vi "Resynchronization Init.vi"(8 "error in":errorcluster, 11 "SCADA in":refnum<class "EMS.lvclass">) -> (0 "error out":errorcluster, 3 "SCADA out":refnum<class "EMS.lvclass">)   [LabVIEW 2018, in "EMS Core.lvlib" / "EMS.lvclass"]
uses:
  EMS.lvclass
  C:/Program Files (x86)/National Instruments/LabVIEW 2018/vi.lib/ActorFramework/Actor/Actor.lvclass
  Controls/Microgrid State.ctl
  EMS.lvclass/EMS.ctl
  <vilib>/ActorFramework/Actor/Actor.lvclass/Actor.ctl
  <vilib>/ActorFramework/Message Enqueuer/Message Enqueuer.lvclass/Message Enqueuer.ctl
  EMS Messages/Return Microgrid State Msg/Return Microgrid State Msg.lvclass/Return Microgrid State Msg.ctl
  <vilib>/ActorFramework/Message Enqueuer/Enqueue.vi
  <vilib>/ActorFramework/Stop Msg/Stop Msg.lvclass
  C:/Program Files (x86)/National Instruments/LabVIEW 2018/vi.lib/ActorFramework/Message/Message.lvclass
  EMS Messages/Return Microgrid State Msg/Return Microgrid State Msg.lvclass
  <vilib>/ActorFramework/Message Priority Queue/Priority Enqueue.vi
  <vilib>/ActorFramework/Actor/Actor.lvclass
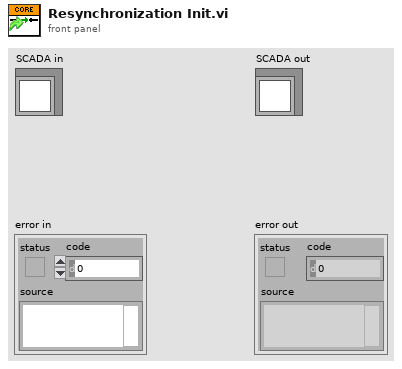
[diagram p1: front panel]
types:
  T1 = typedef "EMS Core.lvlib/EMS.lvclass/Microgrid State.ctl" = enum16{"Discovery", "Commissioning", "Activation", "Blackstart", "OnGrid", "OffGrid", "Island", "Resynchronization", "Manual", "Shutdown", "Stop"}
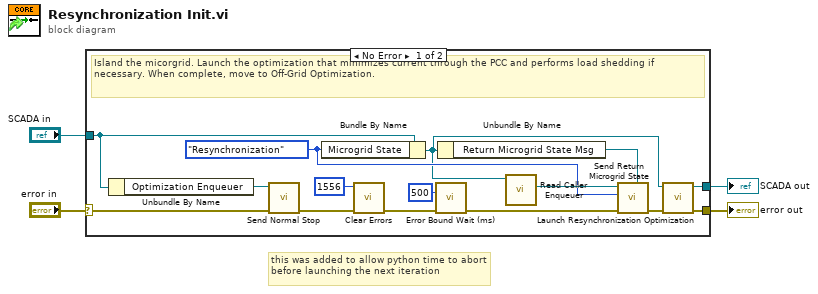
[diagram p0: block diagram]
diagram:
  # "this was added to allow python time to abort before launching the next iteration"
  n1 = case shown="No Error" "error in" {
    selector: "error in" -> [w14 w21]
    tunnel: [w10 w21] -> w3
    tunnel: [w11 w20] -> w1
    tunnel: "SCADA in" -> [w16 w20]
    frame No Error {
      w17 = Microgrid_State."Resynchronization" ("Microgrid State")
      # "Island the micorgrid. Launch the optimization that minimizes current through the PCC and performs load shedding if necessary. When complete, move to Off-Grid Optimization."
      n2 = Unbundle By Name(w16) -> ("Optimization Enqueuer"=w15:refnum<class "Message Enqueuer.lvclass">)
      n3 = call <vilib>:"Send Normal Stop.vi"("error in (no error)"=w14, "Message Enqueuer"=w15) -> ("error out"=w13:errorcluster)  [unwired: 9 in]
      n4 = Bundle By Name(cluster=w16, "Microgrid State"=w17) -> (w12:refnum<class "EMS.lvclass">)
      n5 = call <vilib>:"Clear Errors.vi"("error in (no error)"=w13, "specific error code to clear (0: all)"=1556) -> ("error out"=w8:errorcluster)  [unwired: 4 in, 1 out]
      n6 = call "Error Bound Wait (ms).vi"("milliseconds to wait (100)"=u32 500 ("milliseconds to wait"), "error in"=w8) -> ("error out"=w6:errorcluster)  [unwired: 9 in]
      n7 = Unbundle By Name(w12) -> ("Return Microgrid State Msg"=w18:refnum<class "Return Microgrid State Msg.lvclass">)
      n8 = call <vilib>:"Read Caller Enqueuer.vi"("Actor"=w12) -> ("Caller Enqueuer"=w19:refnum<class "Message Enqueuer.lvclass">)  [unwired: 10 in]
      n9 = call "Send Return Microgrid State.vi"("Message Type"=w18, "error in (no error)"=w6, "Microgrid State"=w17, "Message Enqueuer"=w19) -> ("error out"=w9:errorcluster)  [unwired: 6 in, 1 out]
      n10 = call "Launch Resynchronization Optimization.vi"("error in"=w9, "SCADA in"=w12) -> ("error out"=w10:errorcluster, "SCADA out"=w11:refnum<class "EMS.lvclass">)  [unwired: 8 in]
    }
    frame Error {
    }
  }
  "error out" <- w3
  "SCADA out" <- w1
